vi "ExitGui.vi"() -> (2 "ok":bool, 3 "ExitAction":T1=enum."Log off PC user")   [LabVIEW 2019, in "Tools.lvlib"]
uses:
  Tools.lvlib
  controls/buttons/OK.ctl
  controls/buttons/Cancel.ctl
  Windows/Windows.ExitAction.ctl
  ExitGui.Action.ctl
panel:
  out "_loop":i32(ring)=4
  in  "open?":bool
  in  "ExitOption":u32(ring) items=["Close TMOS", "Log off PC user", "Shut down the computer", "Reboot the computer"]
  in  "CancelButton":T2
  out "Message":string
  in  "OKButton":T3
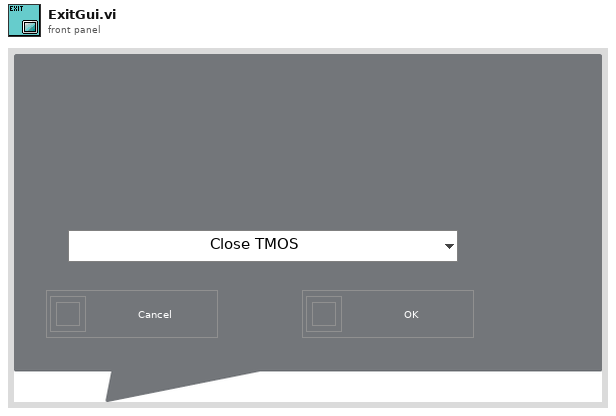
[diagram p1: front panel]
types:
  T1 = typedef "Tools.lvlib/Windows.ExitAction.ctl" = enum16{"Close TMOS", "Log off PC user", "Shut down the computer", "Reboot the computer"}
  T2 = typedef "Tools.lvlib/Cancel.ctl" = bool
  T3 = typedef "Tools.lvlib/OK.ctl" = bool
  T4 = typedef "Tools.lvlib/ExitGui.Action.ctl" = enum32{"idle", "constructor", "destructor", "--- ExitGUI ---", "Gui.Translate"}
  T5 = enum32{"invalid app kind", "Development System", "Run Time System", "Student Edition", "Embedded LabVIEW", "Evaluation", "Custom"}
  T6 = typedef "LVPositionTypeDef.ctl" = cluster{"Left":i32, "Top":i32}
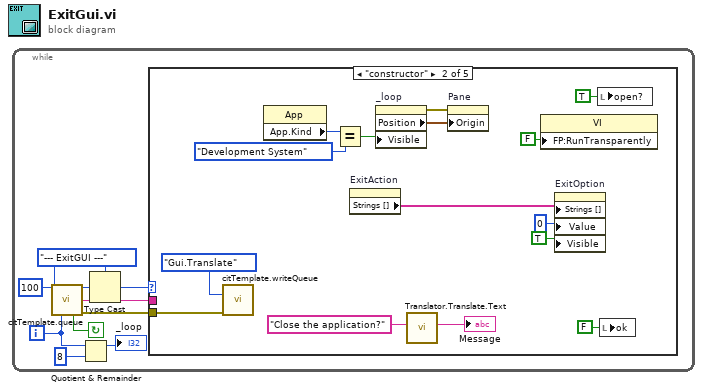
[diagram p0: block diagram]
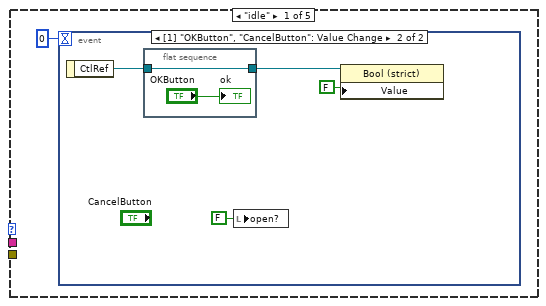
[diagram p2: hidden frame]
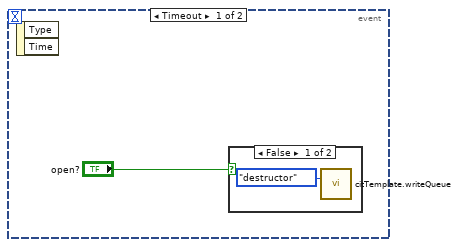
[diagram p3: hidden frame]
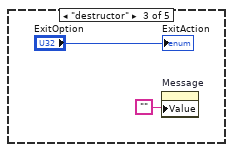
[diagram p5: hidden frame]
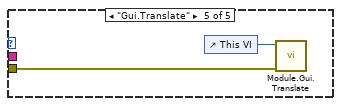
[diagram p7: hidden frame]
diagram:
  n1 = while {
    i -> [w1]
    stop <- w10 continue-if-true
    w4 = ExitGui.Action."--- ExitGUI ---" ("Action")
    n2 = call "citTemplate.queue.vi"("ms timeout (250 ms)"=100, "event enum"=w4, "iteration (-1)"=w1) -> ("event out"=w8:u32, "(flatten) data out"=w5:string, "continue"=w10:bool, "error out"=w6:errorcluster)  [unwired: 2 in, 7 out]
    n3 = Quotient & Remainder(x=w1, y=8) -> (x-y*floor(x/y)=→"_loop":i32)  [unwired: 1 out]
    n4 = Type Cast(type=w4, x=w8) -> (*(type *) &x=w7:T4)
    n5 = case shown="\"constructor\"" w7 {
      tunnel: w6 -> [_ w22 _ _ w37]
      tunnel: w5 -> [_ _ _ _ _]
      frame "idle" {
        n6 = event shown="[1] \"OKButton\", \"CancelButton\": Value Change" {
          selector: _ -> [_ _]
          dyn-events: _ -> [_ _]
          timeout: 0 -> [_ _]
          event Timeout {
            n7 = event-data() -> ()  [unwired: 3 out]
            n8 = case shown="False" "open?" {
              frame False {
                n9 = call "citTemplate.writeQueue.vi"("event in (if not connected:all statemachine with data event)"=ExitGui.Action."destructor" ("Action")) -> ()  [unwired: 4 in, 11 out]
              }
              frame True {
              }
            }
          }
          event Value Change {
            n10 = event-data() -> ("CtlRef"=w15:refnum<vi>)  [unwired: 1 out]
            n11 = flat-sequence {
              tunnel: w15 -> [w18]
              tunnel: [w18] -> w14
              frame #0 {
                "ok" <- "OKButton"
              }
            }
            n12 = local write "open?"(FALSE ("open?")) -> ()
            n13 = property class="Bool (strict)"(reference=w14, "Value"=T2 FALSE) -> ()  [unwired: 1 in, 2 out]
          }
        }
      }
      frame "constructor" {
        n14 = call "citTemplate.writeQueue.vi"("event in (if not connected:all statemachine with data event)"=ExitGui.Action."Gui.Translate" ("Action"), "error in (no error)"=w22) -> ()  [unwired: 13 in, 1 out]
        n15 = property class="App"() -> ("App.Kind"=w29:T5)  [unwired: 2 in, 2 out]
        n16 = Equal?(x=w29, y=T5."Development System") -> (x = y?=w27:bool)
        n17 = property on="ExitAction" class="Enum (strict)"() -> ("Strings []"=w23:string[])  [unwired: 2 in, 2 out]
        n18 = property on="_loop" class="Ring (strict)"("Visible"=w27) -> (error out=w31:errorcluster, "Position"=w32:T6)  [unwired: 2 in, 1 out]
        n19 = call "Translator.Translate.Text.vi"("text"="Close the application?" ("Message")) -> ("translated text"=→"Message":string)  [unwired: 9 in, 1 out]
        n20 = property on="Pane" class="Pane"(error in=w31, "Origin"=w32) -> ()  [unwired: 1 in, 2 out]
        n21 = property class="VI"("FP:RunTransparently"=FALSE ("Front Panel Window:Run VI Transparently")) -> ()  [unwired: 2 in, 2 out]
        n22 = property on="ExitOption" class="Ring (strict)"("Strings []"=w23, "Value"=0 ("length"), "Visible"=TRUE) -> ()  [unwired: 2 in, 2 out]
        n23 = local write "open?"(TRUE ("open?")) -> ()
        n24 = local write "ok"(FALSE ("_b_ok")) -> ()
      }
      frame "destructor" {
        n25 = property on="Message" class="Str"("Value"="") -> ()  [unwired: 2 in, 2 out]
        "ExitAction" <- "ExitOption"
      }
      frame "--- ExitGUI ---" {
      }
      frame "Gui.Translate" {
        n26 = control-ref of="This VI"() -> (w38:refnum<vi>)
        n27 = call "Module.Gui.Translate.vi"("error in"=w37, "VI ref in"=w38) -> ()  [unwired: 7 in, 3 out]
      }
    }
  }
